vi "Get CMMTable106 Clmns.vi"(10 "Column Titles":string[](array[string]), 11 "[[CMM Table 106]]":string[][](array[string])) -> (3 "Columns out":dbl[][](array[numeric]))   [LabVIEW 2018, in "RT - Analysis.lvlib"]
uses:
  RT - Analysis.lvlib
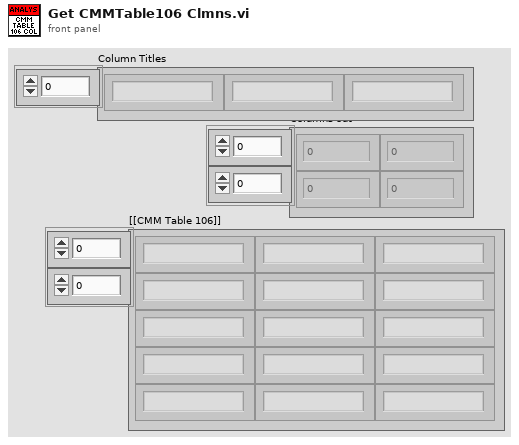
[diagram p1: front panel]
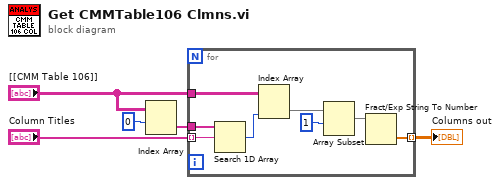
[diagram p0: block diagram]
diagram:
  n1 = Index Array(array="[[CMM Table 106]]", index (row)=0) -> (element=w2:string[])  [unwired: 1 in]
  n2 = for {
    tunnel: w2 -> [w13]
    tunnel: "Column Titles" -> [w12] mode=indexing
    tunnel: "[[CMM Table 106]]" -> [w11]
    tunnel: [w8] -> w5 mode=indexing
    n3 = Search 1D Array(1D array=w13, element=w12) -> (index of element=w10:i32)  [unwired: 1 in]
    n4 = Index Array(array=w11, index (col)=w10) -> (element=w9:string[])  [unwired: 1 in]
    n5 = Array Subset(array=w9, index=1) -> (w7:string[])  [unwired: 1 in]
    n6 = Fract/Exp String To Number(string=w7) -> (number=w8:dbl[])  [unwired: 3 in, 1 out]
  }
  "Columns out" <- w5
